vi "Close Body References.vi"(8 "Error In":errorcluster, 11 "BodyData":T1={"ClippedEdges"=enum."None", "HandLeftConfidence"=enum."High", "HandLeftState"=enum."NotTracked", "HandRightConfidence"=enum."High", "HandRightState"=enum."NotTracked", "IsRestricted"=FALSE, "IsTracked"=FALSE, "JointOrientations"=refnum, "Joints"=refnum, "Lean"=refnum, "LeanTrackingState"=enum."NotTracked", "TrackingId"=0}) -> (0 "Error Out":errorcluster)   [LabVIEW 2011, in "KinectOne.lvlib"]
uses:
  KinectOne.lvlib
  Type Defs/BodyData.ctl
  Type Defs/ClippedEdges.ctl
  Type Defs/HandLeftConfidence.ctl
  Type Defs/HandLeftState.ctl
  Type Defs/HandRightConfidence.ctl
  Type Defs/HandRightState.ctl
  Microsoft.Kinect
  Type Defs/LeanTrackingState.ctl
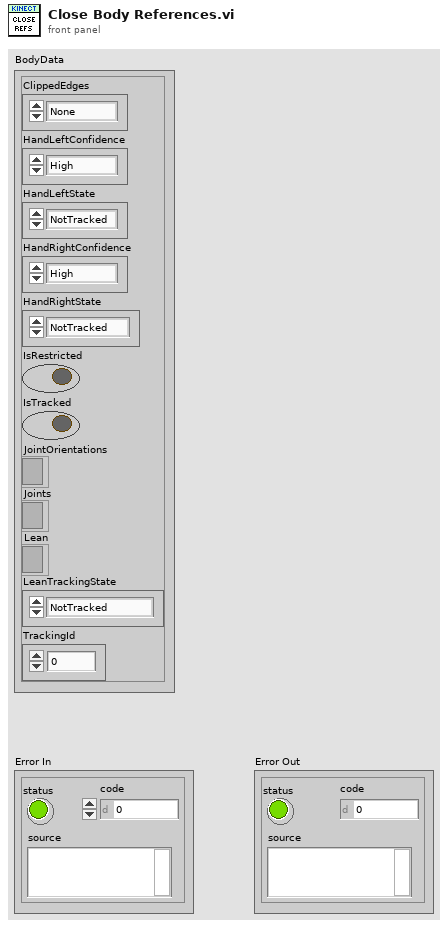
[diagram p1: front panel]
types:
  T1 = typedef "KinectOne.lvlib/BodyData.ctl" = cluster{"ClippedEdges":T2, "HandLeftConfidence":T3, "HandLeftState":T4, "HandRightConfidence":T5, "HandRightState":T6, "IsRestricted":bool, "IsTracked":bool, "JointOrientations":refnum<k24>, "Joints":refnum<k24>, "Lean":refnum<k24>, "LeanTrackingState":T7, "TrackingId":u64}
  T2 = typedef "KinectOne.lvlib/ClippedEdges.ctl" = enum16{"None", "Right", "Left", "Top", "Bottom"}
  T3 = typedef "KinectOne.lvlib/HandLeftConfidence.ctl" = enum16{"Low", "High"}
  T4 = typedef "KinectOne.lvlib/HandLeftState.ctl" = enum16{"Unknown", "NotTracked", "Open", "Closed", "Lasso"}
  T5 = typedef "KinectOne.lvlib/HandRightConfidence.ctl" = enum16{"Low", "High"}
  T6 = typedef "KinectOne.lvlib/HandRightState.ctl" = enum16{"Unknown", "NotTracked", "Open", "Closed", "Lasso"}
  T7 = typedef "KinectOne.lvlib/LeanTrackingState.ctl" = enum16{"NotTracked", "Inferred", "Tracked"}
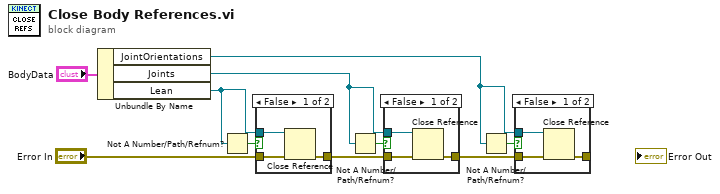
[diagram p0: block diagram]
diagram:
  n1 = Unbundle By Name("BodyData") -> ("JointOrientations"=w1:refnum<k24>, "Joints"=w4:refnum<k24>, "Lean"=w8:refnum<k24>)
  n2 = Not A Number/Path/Refnum?(number/path/refnum=w8) -> (NaN/Path/Refnum?=w7:bool)
  n3 = case shown="False" w7 {
    tunnel: [w13 w14] -> w5
    tunnel: "Error In" -> [w12 w14]
    tunnel: w8 -> [w11 _]
    frame False {
      n4 = Close Reference(reference=w11, error in (no error)=w12) -> (error out=w13:errorcluster)
    }
    frame True {
    }
  }
  n5 = Not A Number/Path/Refnum?(number/path/refnum=w4) -> (NaN/Path/Refnum?=w6:bool)
  n6 = case shown="False" w6 {
    tunnel: [w17 w18] -> w2
    tunnel: w5 -> [w16 w18]
    tunnel: w4 -> [w15 _]
    frame False {
      n7 = Close Reference(reference=w15, error in (no error)=w16) -> (error out=w17:errorcluster)
    }
    frame True {
    }
  }
  n8 = Not A Number/Path/Refnum?(number/path/refnum=w1) -> (NaN/Path/Refnum?=w3:bool)
  n9 = case shown="False" w3 {
    tunnel: [w21 w22] -> _
    tunnel: w2 -> [w20 w22]
    tunnel: w1 -> [w19 _]
    frame False {
      n10 = Close Reference(reference=w19, error in (no error)=w20) -> (error out=w21:errorcluster)
    }
    frame True {
    }
  }
